vi "OE1022_Query Data.vi"(0 "VISA resource name":refnum<visa-resource-name>, 7 "Remote Mode":u16(ring) items=["USB"=0, "GPIB"=2], 9 "Timeout":u32=1000, 11 "Error in (no error)":errorcluster caption="error out（no error）") -> (4 "VISA resource  out":refnum<visa-resource-name>, 6 "Parameter Values":T1, 8 "Data Array":dbl[](array[numeric]), 10 "Output String":string, 15 "Error out":errorcluster caption="error out")   [LabVIEW 2011]
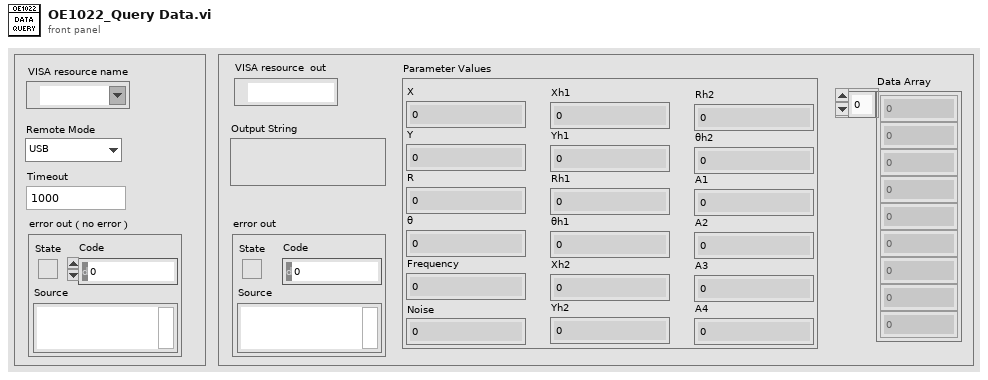
[diagram p1: front panel]
types:
  T1 = cluster{"X":dbl, "Y":dbl, "R":dbl, "θ":dbl, "Frequency":dbl, "Xh1":dbl, "Yh1":dbl, "Rh1":dbl, "θh1":dbl, "Xh2":dbl, "Yh2":dbl, "Rh2":dbl, "θh2":dbl, "Noise":dbl, "A1":dbl, "A2":dbl, "A3":dbl, "A4":dbl}
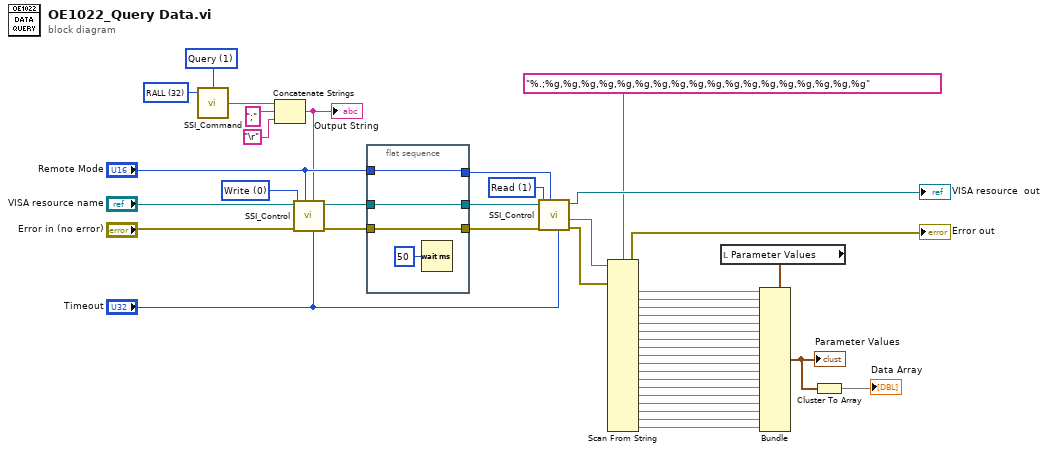
[diagram p0: block diagram]
diagram:
  w6 = u16 32 items=["ISRC", "IGND", "ICPL", "ILIN", "PHAS", "FMOD", "RSLP", "FREQ", "SWPT", "SLLM", "SULM", "SSLL", "SSLG", "STLM", "SWRM", "IRNG", "SENS", "RMOD", "OFLT", "OFSL", "SYNC", "DMOD", "HARM", "DARB", "SWVT", "SLVL", "SVLL", "SVUL", "SVSL", "SVSG", "SVTM", "SVRM", "RALL", "SNAP", "OUTP", "OAUX", "COUT", "CAUX", "COFP", "CEXP", "FPOP", "OEXP", "*IDN", "*RST", "OVLD", "INOV", "GNOV", "*PLL", "SSET", "RSET", "AGAN", "APHS", "ARSV", "ASCL", "EQCD", "EQCS", "SPED", "SRAT", "SLEN", "SSLE", "STRG", "SPRM", "STRD", "PAUS", "RSET", "SPTS", "TRCA", "TEMP", "RSTU", "INHZ", "DEQU", "SADD", "ARNG", "CSPE", "ISRCD", "IGNDD", "ICPLD", "ILIND", "PHASD", "FMODD", "RSLPD", "FREQD", "SWPTD", "SLLMD", "SULMD", "SSLLD", "SSLGD", "STLMD", "SWRMD", "SENSD", "RMODD", "OFLTD", "OFSLD", "SYNCD", "HARMD", "EQCDD", "EQCSD", "SNAPD", "OUTPD", "SWVTD", "SLVLD", "SVLLD", "SVULD", "SVSLD", "SVSGD", "SVTMD", "SVRMD", "SVDCD", "ARSVD", "AGAND", "APHSD", "ASCLD", "FPOPD", "CAUXD", "OEXPD", "SPEDD", "SRATD", "SLEND", "SSLED", "STRGD", "SPRMD", "STRDD", "PAUSD", "RESTD", "SPTSD", "TRCAD", "*IDND", "*RSTD", "INOVD", "GNOVD", "*PLLD", "SSETD", "RSETD", "RALLD"] ("Command Type")
  w33 = u16 1 items=["Write", "Read"] ("Control")
  w38 = u16 1 items=["Set", "Query"] ("Opera")
  w39 = u16 0 items=["Write", "Read"] ("Control")
  n1 = call "SSI_Command.vi"("Opera"=w38, "Command Type"=w6) -> ("Output string"=w4:string)  [unwired: 2 in]
  n2 = Concatenate Strings(w4, ";" ("字符串"), "\r") -> (w31:string)
  "Output String" <- w31
  n3 = call "SSI_Control.vi"("Tineout"="Timeout", "Write Buffer"=w31, "Remote Mode"="Remote Mode", "Error in (no error)"="Error in (no error)", "Control"=w39, "VISA resource name"="VISA resource name") -> ("Error out"=w36:errorcluster, "VISA resource  out"=w37:refnum<visa-resource-name>)  [unwired: 2 in, 2 out]
  n4 = flat-sequence {
    tunnel: w37 -> [w47]
    tunnel: w36 -> [w46]
    tunnel: [w47] -> w35
    tunnel: [w46] -> w34
    tunnel: [w44] -> w32
    tunnel: "Remote Mode" -> [w44]
    frame #0 {
      n5 = Wait (ms)(milliseconds to wait=u32 50 ("等待时间（毫秒）")) -> ()  [unwired: 1 out]
    }
  }
  n6 = call "SSI_Control.vi"("Tineout"="Timeout", "Remote Mode"=w32, "Error in (no error)"=w34, "Control"=w33, "VISA resource name"=w35) -> ("Error out"=w29:errorcluster, "Read Buffer"=w30:string, "VISA resource  out"=→"VISA resource  out":refnum<visa-resource-name>)  [unwired: 3 in, 1 out]
  n7 = Scan From String(format string="%.;%g,%g,%g,%g,%g,%g,%g,%g,%g,%g,%g,%g,%g,%g,%g,%g,%g,%g" ("格式字符串"), input string=w30, error in=w29) -> (error out=→"Error out":errorcluster, output 1=w27:dbl, output 2=w26:dbl, output 3=w25:dbl, output 4=w24:dbl, output 5=w23:dbl, output 6=w19:dbl, output 7=w18:dbl, output 8=w17:dbl, output 9=w16:dbl, output 10=w15:dbl, output 11=w14:dbl, output 12=w13:dbl, output 13=w12:dbl, output 14=w11:dbl, output 15=w10:dbl, output 16=w9:dbl, output 17=w8:dbl, output 18=w7:dbl)  [unwired: 19 in, 2 out]
  n8 = local read "Parameter Values"() -> (w21:T1)
  n9 = Bundle(cluster=w21, "X"=w27, "Y"=w26, "R"=w25, "θ"=w24, "Frequency"=w23, "Xh1"=w19, "Yh1"=w18, "Rh1"=w17, "θh1"=w16, "Xh2"=w15, "Yh2"=w14, "Rh2"=w13, "θh2"=w12, "Noise"=w11, "A1"=w10, "A2"=w9, "A3"=w8, "A4"=w7) -> (w2:T1)
  "Parameter Values" <- w2
  n10 = Cluster To Array(cluster=w2) -> (array=→"Data Array":dbl[])
